vi "Set Write Timeout.vi"(8 "error in (no error)":errorcluster, 10 "write operation timeout":i32=5000, 11 "Modbus master in":refnum<class "ELAN Master.lvclass">) -> (0 "error out":errorcluster, 3 "Modbus master out":refnum<class "ELAN Master.lvclass">)   [LabVIEW 2021, in "ELAN Master.lvclass"]
doc: "<B>Write Timeout</B> specifies the write operation timeout. You can use a Modbus master instance to perform write operations on a Modbus slave with the specified timeout."
uses:
  ELAN Master.lvclass
  ELAN Master.lvclass/ELAN Master.ctl
  Transmission Data Unit/ELAN/ELAN Data Unit.lvclass/ELAN Data Unit.ctl
  Transmission Data Unit/ELAN/ELAN Data Unit.lvclass
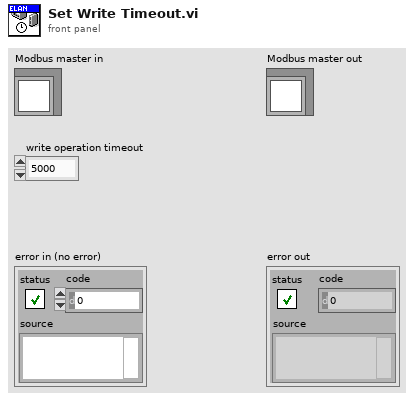
[diagram p1: front panel]
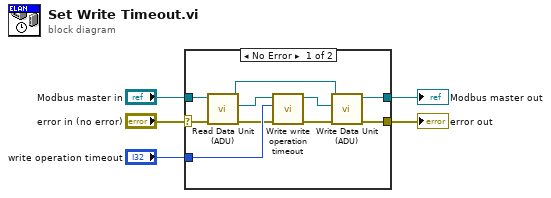
[diagram p0: block diagram]
diagram:
  n1 = case shown="No Error" "error in (no error)" {
    selector: "error in (no error)" -> [w6 w17]
    tunnel: "write operation timeout" -> [w12 _]
    tunnel: "Modbus master in" -> [w11 w16]
    tunnel: [w10 w16] -> w3
    tunnel: [w9 w17] -> w2
    frame No Error {
      n2 = call "Read Data Unit (ADU).vi"("error in (no error)"=w6, "ELAN Master in"=w11) -> ("error out"=w7:errorcluster, "ASCII Data Unit"=w13:refnum<class "ELAN Data Unit.lvclass">, "ELAN Master out"=w15:refnum<class "ELAN Master.lvclass">)  [unwired: 7 in]
      n3 = call "Write write operation timeout.vi"("error in (no error)"=w7, "write operation timeout"=w12, "ELAN Data Unit in"=w13) -> ("error out"=w8:errorcluster, "ELAN Data Unit out"=w14:refnum<class "ELAN Data Unit.lvclass">)  [unwired: 7 in]
      n4 = call "Write Data Unit (ADU).vi"("error in (no error)"=w8, "ASCII Data Unit"=w14, "ELAN Master in"=w15) -> ("error out"=w9:errorcluster, "ELAN Master out"=w10:refnum<class "ELAN Master.lvclass">)  [unwired: 7 in]
    }
    frame Error {
    }
  }
  "error out" <- w2
  "Modbus master out" <- w3
